vi "WPI_IMU_FGV.vi"(0 "SimpleGyroDevRef":T3={"DevStatus"={"status"=FALSE, "code"=0, "source"=""}, "Handle"=0, "SPI Bus"=enum."SPI On-Board, CS0", "Device Found"=FALSE, "Sample Rate"=0.0, "Device Ready"=FALSE, "Yaw Axis"=enum."Z"} {"Sample Rate" min=0.25 max=100.0 step=0.25}, 1 "Operation":enum16{"set", "get"}(ring), 2 "Sensor Ready?":bool, 5 "Reset":bool, 7 "IMU Data":T2, 9 "IMU Angles":T1, 11 "IMU AHRS":cluster{"Pitch":dbl, "Roll":dbl, "Yaw":dbl}, 12 "IMU AHRS DELTA":cluster{"Pitch":dbl, "Roll":dbl, "Yaw":dbl}) -> (4 "SimpleGyroDevRef":T3={"DevStatus"={"status"=FALSE, "code"=0, "source"=""}, "Handle"=0, "SPI Bus"=enum."SPI On-Board, CS0", "Device Found"=FALSE, "Sample Rate"=0.0, "Device Ready"=FALSE, "Yaw Axis"=enum."Z"} {"Sample Rate" min=0.25 max=100.0 step=0.25}, 6 "Reset Out":bool, 8 "IMU Data Out":T2, 10 "IMU Angles Out":T1, 13 "Sensor Ready Out":bool, 14 "IMU AHRS DELTA Out":cluster{"Pitch":dbl, "Roll":dbl, "Yaw":dbl}, 15 "IMU AHRS Out":cluster{"Pitch":dbl, "Roll":dbl, "Yaw":dbl})   [LabVIEW 2015, in "FRC ADI MXP IMU.lvlib"]
uses:
  FRC ADI MXP IMU.lvlib
  WPI_AnalogDevicesIMUDevRef.ctl
  <vilib>/Rock Robotics/SystemInterfaces/spilib/spi_bus.ctl
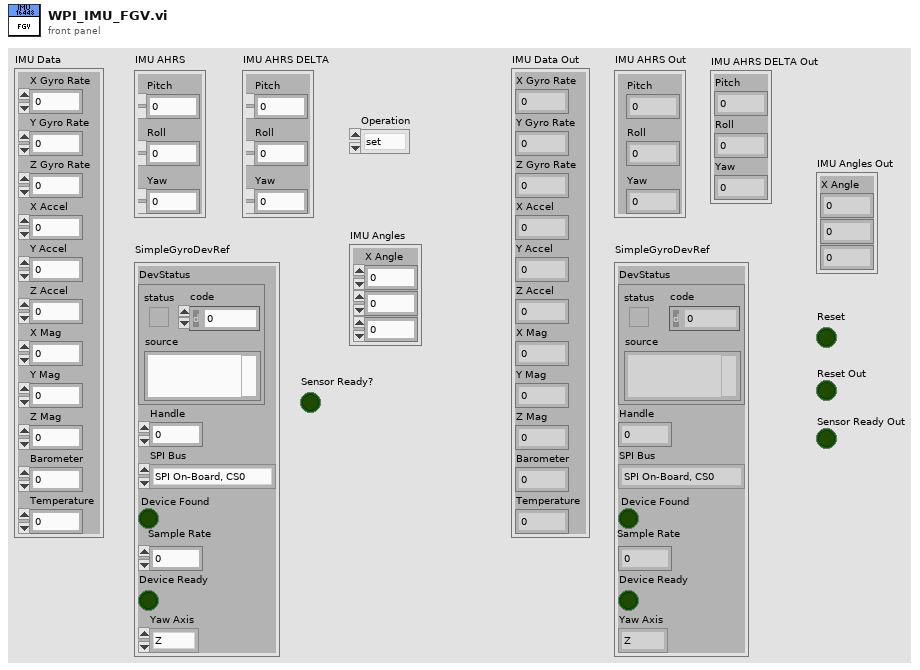
[diagram p1: front panel]
types:
  T1 = cluster{"X Angle":dbl, "Y Angle":dbl, "Z Angle":dbl}
  T2 = cluster{"X Gyro Rate":dbl, "Y Gyro Rate":dbl, "Z Gyro Rate":dbl, "X Accel":dbl, "Y Accel":dbl, "Z Accel":dbl, "X Mag":dbl, "Y Mag":dbl, "Z Mag":dbl, "Barometer":dbl, "Temperature":dbl}
  T3 = typedef "FRC ADI MXP IMU.lvlib/WPI_AnalogDevicesIMUDevRef.ctl" = cluster{"DevStatus":errorcluster, "Handle":i32, "SPI Bus":T4, "Device Found":bool, "Sample Rate":dbl, "Device Ready":bool, "Yaw Axis":enum16{"X", "Y", "Z"}}
  T4 = typedef "spi_bus.ctl" = enum16{"SPI On-Board, CS0", "SPI On-Board, CS1", "SPI On-Board, CS2", "SPI On-Board, CS3", "SPI MXP", "Invalid"}
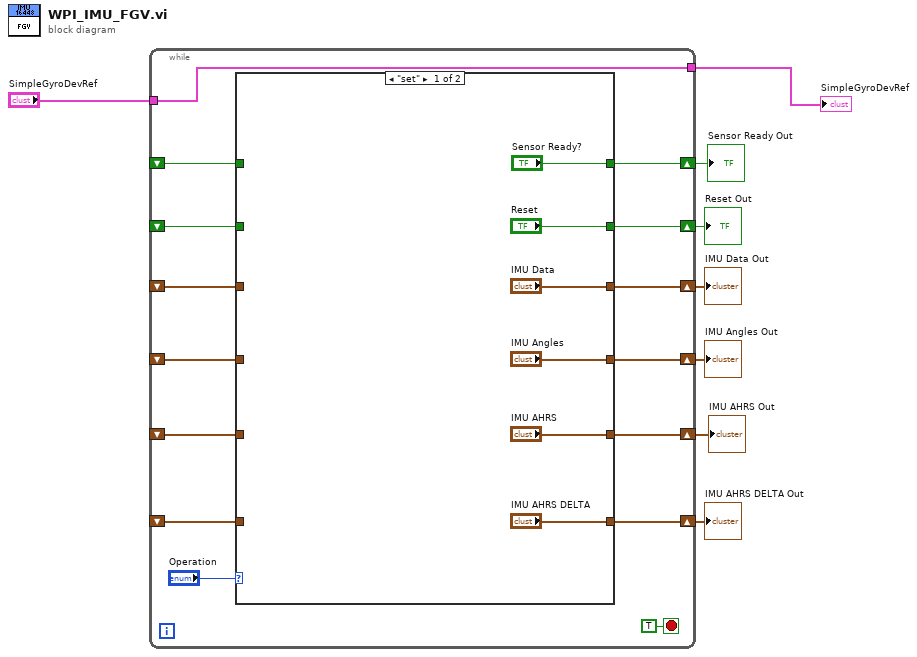
[diagram p0: block diagram]
diagram:
  n1 = while {
    shift-right: [w21] -> w5
    shift-left: _ -> [w15]
    shift-right: [w20] -> w6
    shift-left: _ -> [w16]
    tunnel: "SimpleGyroDevRef" -> [w19]
    tunnel: [w19] -> w7
    shift-right: [w18] -> w4
    shift-left: _ -> [w17]
    shift-right: [w14] -> w3
    shift-left: _ -> [w13]
    shift-right: [w12] -> w2
    shift-left: _ -> [w11]
    shift-right: [w10] -> w1
    shift-left: _ -> [w9]
    stop <- TRUE stop-if-true
    n2 = case shown="\"set\"" "Operation" {
      tunnel: ["Reset" w33] -> w21
      tunnel: ["IMU Data" w34] -> w20
      tunnel: ["IMU Angles" w35] -> w18
      tunnel: w17 -> [_ w35]
      tunnel: w16 -> [_ w34]
      tunnel: w15 -> [_ w33]
      tunnel: ["IMU AHRS" w32] -> w14
      tunnel: w13 -> [_ w32]
      tunnel: ["IMU AHRS DELTA" w31] -> w12
      tunnel: w11 -> [_ w31]
      tunnel: ["Sensor Ready?" w30] -> w10
      tunnel: w9 -> [_ w30]
      frame "set" {
      }
      frame "get", Default {
      }
    }
  }
  "SimpleGyroDevRef" <- w7
  "IMU Data Out" <- w6
  "Reset Out" <- w5
  "IMU Angles Out" <- w4
  "IMU AHRS Out" <- w3
  "IMU AHRS DELTA Out" <- w2
  "Sensor Ready Out" <- w1
